vi "LoadDAQSettings.vi"(2 "error in":errorcluster, 4 "Current ExpState IN":T5={"error"={"status"=FALSE, "code"=0, "source"=""}, "Digitizer DAQmx Tasks"={"TaskArray"=[]}, "DAQ Settings"={"Channel Settings"=[], "Card Settings"=[]}, "Synchronization Settings"={"Synchronizer 0"="", "source terminal"="", "Synchronizer 1"="PXI1Slot2"}, "DAQ Data"=[], "Next Shot#"="", "System Message"="", "User Shot Notes"="", "Timing Settings"={"Timing Card Settings"=[], "Timing Channel Settings"=[]}, "Timing Tasks"={"TaskArray"=[]}, "Tree"="", "Time Card/Channels"=[2, 8], "DAQ Card/Channels"=[3, 8], "Program Version"="", "RIO Settings"={"Channel Settings"=[], "Card Settings"=[]}, "RIO References"={"Reference Array"=[]}, "RIO Data"={"RIO Deleaved Data"=[], "Raw Readout"=[]}, "RIO Card/Channels"=[3, 8], "DIO Channels"=0, "DIO Settings"={"DIO Channel Array"=[]}, "Tachometer Controls"={"Tach Calibration folder"=path "Z:/Data/Calibration/Tachometer", "PSU2 charging Voltage [kV]"=0.0, "PSU2 Counter"="", "PSU2 task"="PSU2", "PSU3 Counter"="", "PSU3 task"="", "PSU3 charging Voltage [kV]"=0.0}, "Global Settings"={"Initial Background Values"={"Reference Shot #"=0.0, "Background pressure [Torr]"=0.0, "Cryo temp [V]"=0.0, "Cryo temp [K]"=0.0, "Cryotemp Calibration File"=path ""}, "Gas Puffing"={"Gas A type"="N", "Gas B type"="N", "Gas C type"="N", "Gas A pressure [psi]"=0.0, "Gas B pressure [psi]"=0.0, "Gas C pressure [psi]"=0.0, "Innner Electrode"="", "Middle Electrode"="", "Outer Electrode"="", "Gas A bottle pressure [psi]"=0.0, "Gas B bottle pressure [psi]"=0.0, "Gas C bottle pressure [psi]"=0.0}, "PSU Voltages"={"Bias1 Voltage [V]"=0.0, "Bias2 Voltage [V]"=0.0, "PSU1 Voltage [V]"=0.0, "Puff-PSU1 CH1 Voltage [V]"=0.0, "Puff-PSU1 CH2 Voltage [V]"=0.0, "Puff-PSU1 CH3 Voltage [V]"=0.0}, "Scope Details"={"CH1"="", "CH2"="", "CH3"="", "CH4"="", "CH1 Ground State"="Grounded", "CH2 Ground State"="Grounded", "CH3 Ground State"="Grounded", "CH4 Ground State"="Grounded"}}, "Calibrations"={"CryoTemp"={"Comment"="", "X"=[], "Y"=[]}, "PSU2 Tach"={"Comment"="", "X"=[], "Y"=[]}, "PSU3 Tach"={"Comment"="", "X"=[], "Y"=[]}}} {"Global Settings"."Initial Background Values"."Cryo temp [K]" format="%#_4g"; "RIO Settings"."Card Settings"."Sample Rate" format="%#_3p"; "Timing Settings"."Timing Channel Settings"."FrontPanelTime" format="%.3p"; "Timing Settings"."Timing Channel Settings"."Pulse width (s)" format="%.3p"; "Timing Settings"."Timing Channel Settings"."Delay (s)" format="%.3p"; "DAQ Settings"."Card Settings"."Global Edge Type" items=["Rising"=10280, "Falling"=10171]; "DAQ Settings"."Card Settings"."Sample Rate" format="%#_3p"}, 5 "Tree DVR In":refnum<data-value>) -> (0 "error out":errorcluster, 1 "Digitizer Settings":T4 {"Card Settings"."Global Edge Type" items=["Rising"=10280, "Falling"=10171]; "Card Settings"."Sample Rate" format="%#_3p"})   [LabVIEW 2014]
uses:
  Controls/ExperimentStateCluster.ctl
  Controls/DigitizerSettingsChannelSettings.ctl
  Controls/DigitizerSettingsCardSettingsArray.ctl
  Controls/DigitizerSettingsCardSettings.ctl
  Controls/TimingSettings.ctl
  Controls/TimingCardSettings.ctl
  Controls/TimingChannelSettings.ctl
  Controls/RIOSettingsExperimentStateCluster.ctl
  Controls/RIOChannelSettingsArrayExperimentStateCluster.ctl
  Controls/RIOSettingsChannelSettings.ctl
  Controls/RIOSettingsCardSettingsArray.ctl
  Controls/RIOSettingsCardSettings.ctl
  <vilib>/userdefined/High Color/nirio_resource_hc.ctl
  Controls/RIOData.ctl
  Controls/DIOChannel.ctl
  Controls/TachometerControls.ctl
  Controls/Global Settings/GlobalSettings.ctl
  Controls/Global Settings/InitialBackgroundValues.ctl
  Controls/Global Settings/GasPuffing.ctl
  Controls/Global Settings/PSUVoltages.ctl
  Controls/Global Settings/ScopeDetails.ctl
  Controls/Calibrations/Calibrations.ctl
  Controls/Calibrations/CryoTemoCalibration.ctl
  Controls/Calibrations/PSU2TachCalibration.ctl
  Controls/Calibrations/PSU3TachCalibration.ctl
  <vilib>/MDSplus/Classes/Tree_Class/Tree.lvclass
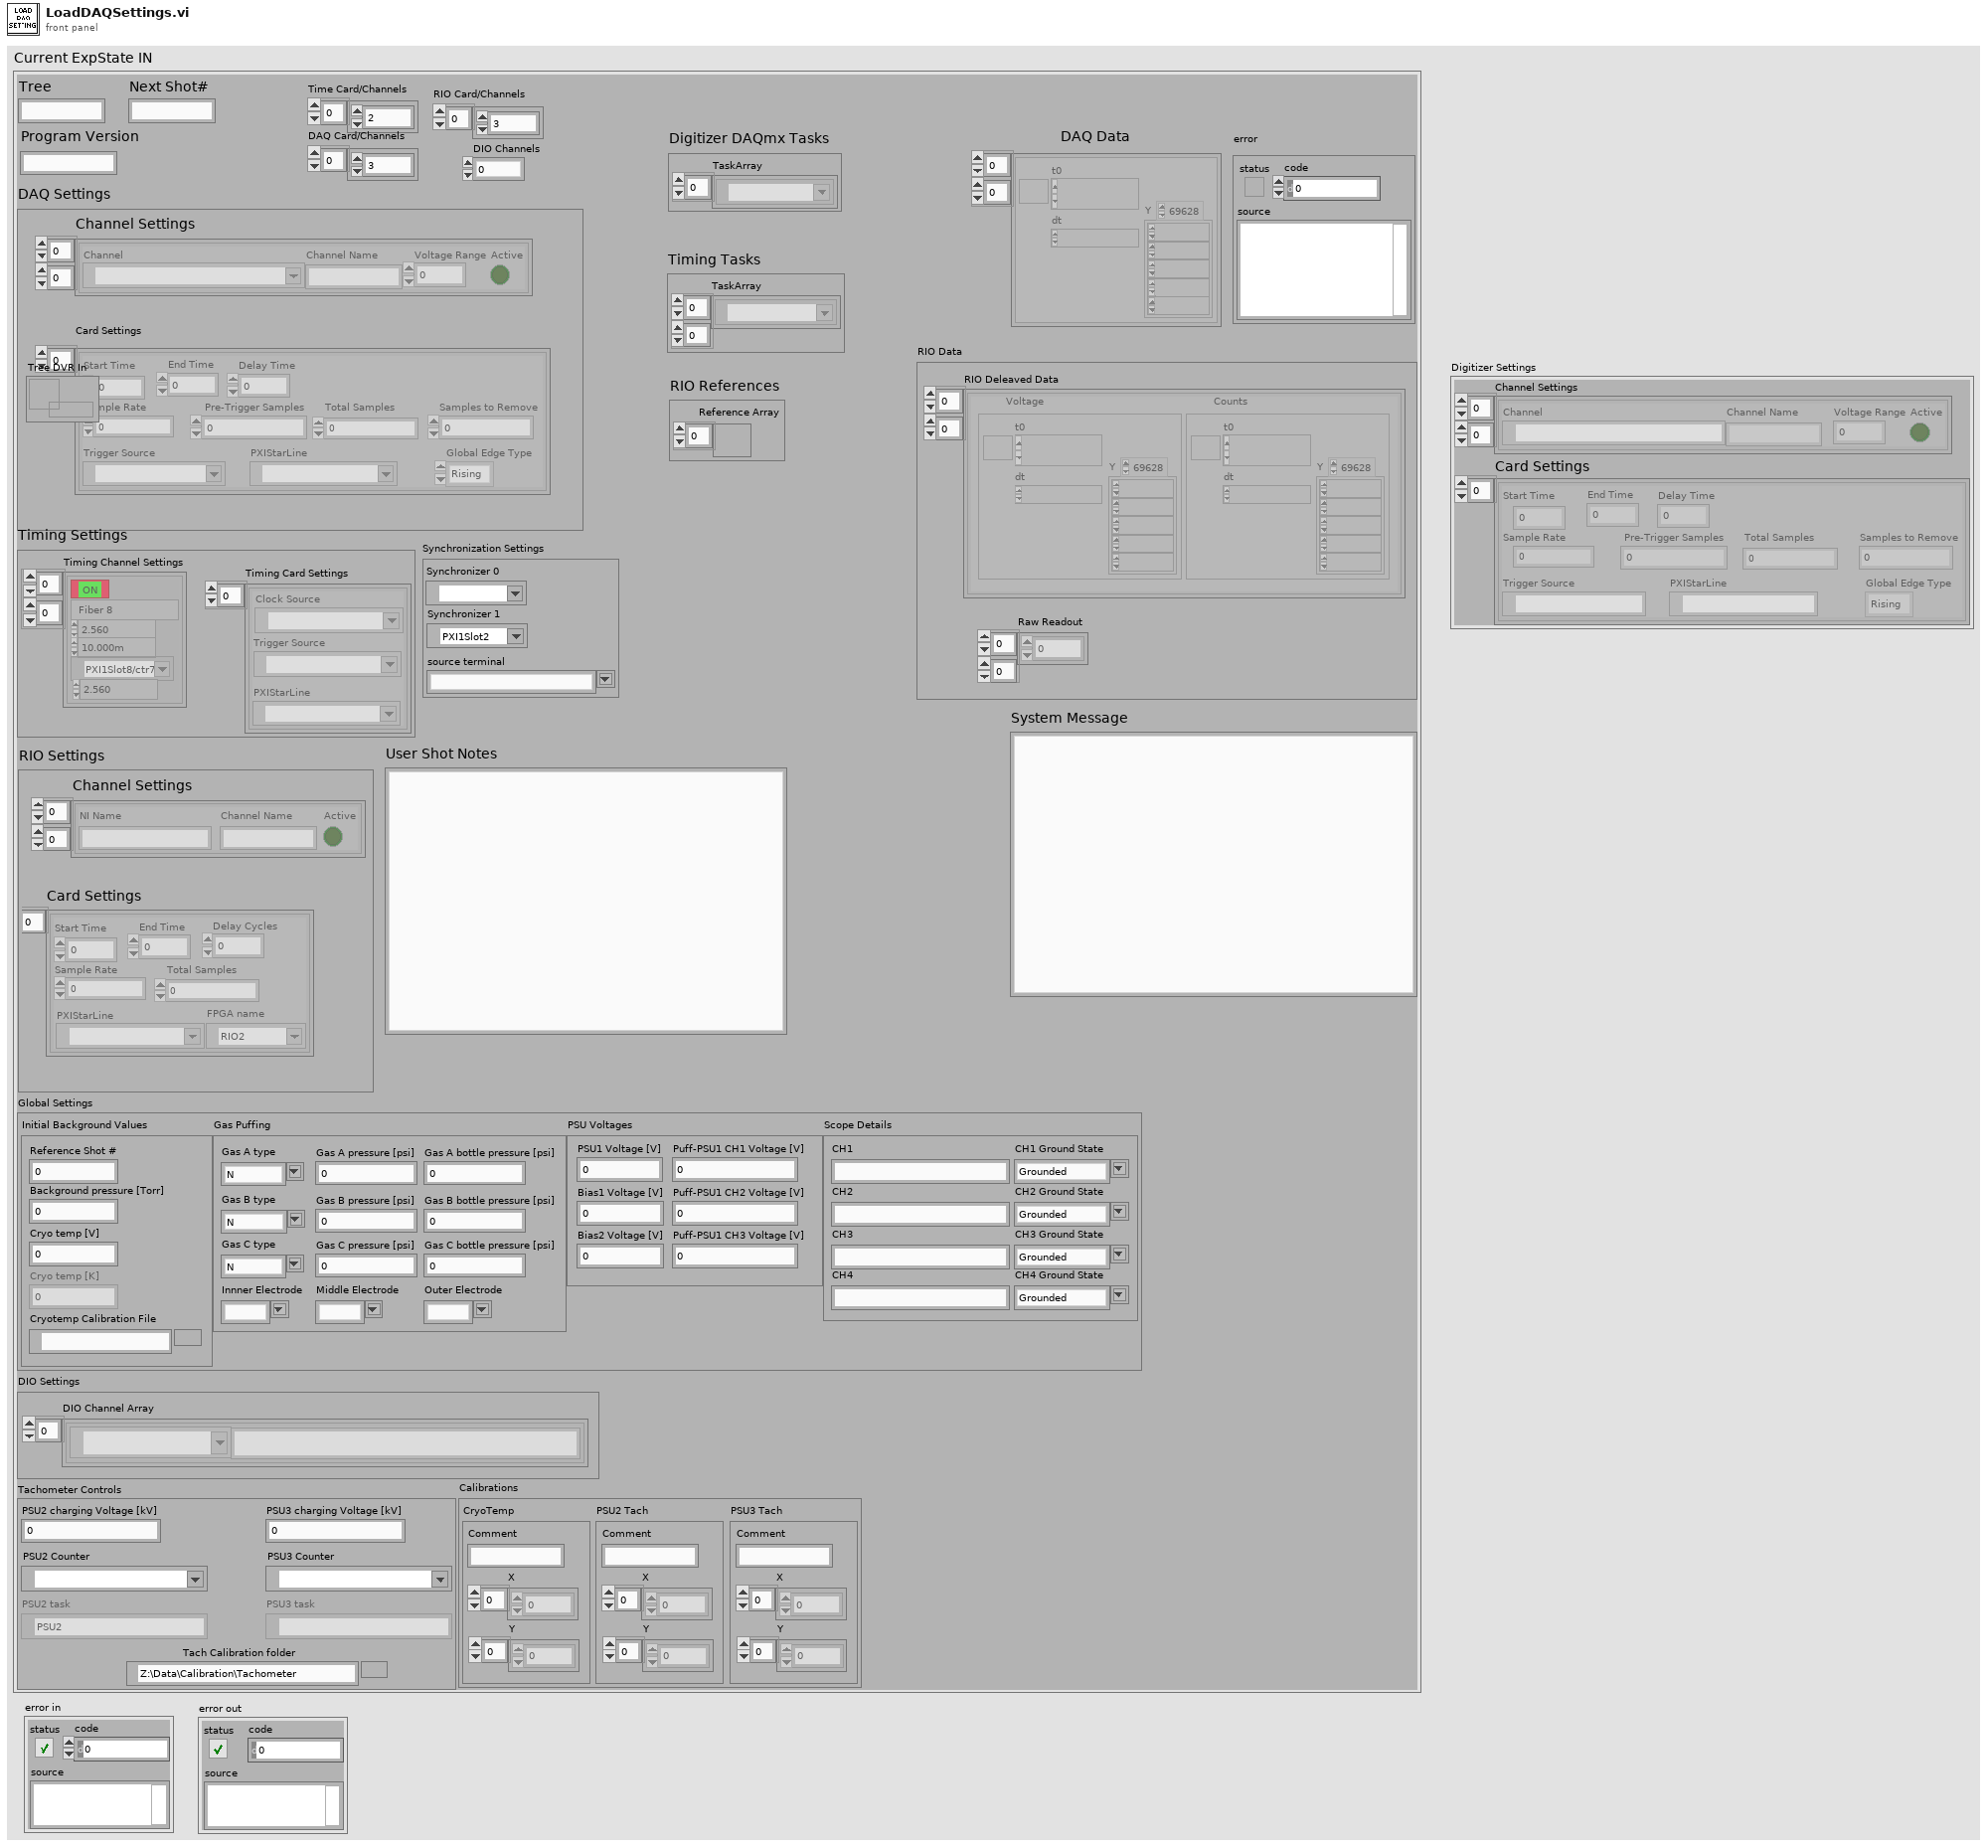
[diagram p1: front panel]
types:
  T1 = typedef "DigitizerSettingsChannelSettings.ctl" = cluster{"Channel":tag, "Channel Name":string, "Voltage Range":dbl, "Active":bool}
  T2 = typedef "DigitizerSettingsCardSettingsArray.ctl" = T3[]
  T3 = typedef "DigitizerSettingsCardSettings.ctl" = cluster{"Start Time":dbl, "End Time":dbl, "Sample Rate":dbl, " Pre-Trigger Samples":u32, "Total Samples":i32, "Samples to Remove":u32, "Trigger Source":tag, "Global Edge Type":i32, "PXIStarLine":tag, "Delay Time":dbl}
  T4 = cluster{"Channel Settings":T1[][], "Card Settings":T2}
  T5 = typedef "ExperimentStateCluster.ctl" = cluster{"error":errorcluster, "Digitizer DAQmx Tasks":cluster{"TaskArray":refnum<k21>[]}, "DAQ Settings":cluster{"Channel Settings":T1[][], "Card Settings":T2}, "Synchronization Settings":cluster{"Synchronizer 0":refnum<k15>, "source terminal":string, "Synchronizer 1":refnum<k15>}, "DAQ Data":waveform(dbl)[][], "Next Shot#":string, "System Message":string, "User Shot Notes":string, "Timing Settings":T6, "Timing Tasks":cluster{"TaskArray":refnum<k21>[][]}, "Tree":string, "Time Card/Channels":i32[], "DAQ Card/Channels":i32[], "Program Version":string, "RIO Settings":T9, "RIO References":cluster{"Reference Array":refnum<k20>[]}, "RIO Data":T15, "RIO Card/Channels":i32[], "DIO Channels":i32, "DIO Settings":cluster{"DIO Channel Array":T16[]}, "Tachometer Controls":T17, "Global Settings":T18, "Calibrations":T23}
  T6 = typedef "TimingSettings.ctl" = cluster{"Timing Card Settings":T7[], "Timing Channel Settings":T8[][]}
  T7 = typedef "TimingCardSettings.ctl" = cluster{"Trigger Source":tag, "Clock Source":tag, "PXIStarLine":tag}
  T8 = typedef "TimingChannelSettings.ctl" = cluster{"Delay (s)":dbl, "Pulse width (s)":dbl, "Active":bool, "Channel Name":string, "counter":tag, "FrontPanelTime":dbl}
  T9 = typedef "RIOSettingsExperimentStateCluster.ctl" = cluster{"Channel Settings":T10, "Card Settings":T12}
  T10 = typedef "RIOChannelSettingsArrayExperimentStateCluster.ctl" = T11[][]
  T11 = typedef "RIOSettingsChannelSettings.ctl" = cluster{"Channel Name":string, "Active":bool, "NI Name":string}
  T12 = typedef "RIOSettingsCardSettingsArray.ctl" = T13[]
  T13 = typedef "RIOSettingsCardSettings.ctl" = cluster{"Start Time":dbl, "End Time":dbl, "Sample Rate":dbl, "Total Samples":u64, "PXIStarLine":tag, "Delay Cycles":u64, "FPGA name":T14}
  T14 = typedef "nirio_resource_hc.ctl" = tag
  T15 = typedef "RIOData.ctl" = cluster{"RIO Deleaved Data":cluster{"Voltage":waveform(dbl), "Counts":waveform(i16)}[][], "Raw Readout":u64[][]}
  T16 = typedef "DIOChannel.ctl" = cluster{"Channel Name":string, "NI Name":tag}
  T17 = typedef "TachometerControls.ctl" = cluster{"Tach Calibration folder":path, "PSU2 charging Voltage [kV]":dbl, "PSU2 Counter":tag, "PSU2 task":refnum<k21>, "PSU3 Counter":tag, "PSU3 task":refnum<k21>, "PSU3 charging Voltage [kV]":dbl}
  T18 = typedef "GlobalSettings.ctl" = cluster{"Initial Background Values":T19, "Gas Puffing":T20, "PSU Voltages":T21, "Scope Details":T22}
  T19 = typedef "InitialBackgroundValues.ctl" = cluster{"Reference Shot #":dbl, "Background pressure [Torr]":dbl, "Cryo temp [V]":dbl, "Cryo temp [K]":dbl, "Cryotemp Calibration File":path}
  T20 = typedef "GasPuffing.ctl" = cluster{"Gas A type":string, "Gas B type":string, "Gas C type":string, "Gas A pressure [psi]":dbl, "Gas B pressure [psi]":dbl, "Gas C pressure [psi]":dbl, "Innner Electrode":string, "Middle Electrode":string, "Outer Electrode":string, "Gas A bottle pressure [psi]":dbl, "Gas B bottle pressure [psi]":dbl, "Gas C bottle pressure [psi]":dbl}
  T21 = typedef "PSUVoltages.ctl" = cluster{"Bias1 Voltage [V]":dbl, "Bias2 Voltage [V]":dbl, "PSU1 Voltage [V]":dbl, "Puff-PSU1 CH1 Voltage [V]":dbl, "Puff-PSU1 CH2 Voltage [V]":dbl, "Puff-PSU1 CH3 Voltage [V]":dbl}
  T22 = typedef "ScopeDetails.ctl" = cluster{"CH1":string, "CH2":string, "CH3":string, "CH4":string, "CH1 Ground State":string, "CH2 Ground State":string, "CH3 Ground State":string, "CH4 Ground State":string}
  T23 = typedef "Calibrations.ctl" = cluster{"CryoTemp":T24, "PSU2 Tach":T25, "PSU3 Tach":T26}
  T24 = typedef "CryoTemoCalibration.ctl" = cluster{"Comment":string, "X":dbl[], "Y":dbl[]}
  T25 = typedef "PSU2TachCalibration.ctl" = cluster{"Comment":string, "X":dbl[], "Y":dbl[]}
  T26 = typedef "PSU3TachCalibration.ctl" = cluster{"Comment":string, "X":dbl[], "Y":dbl[]}
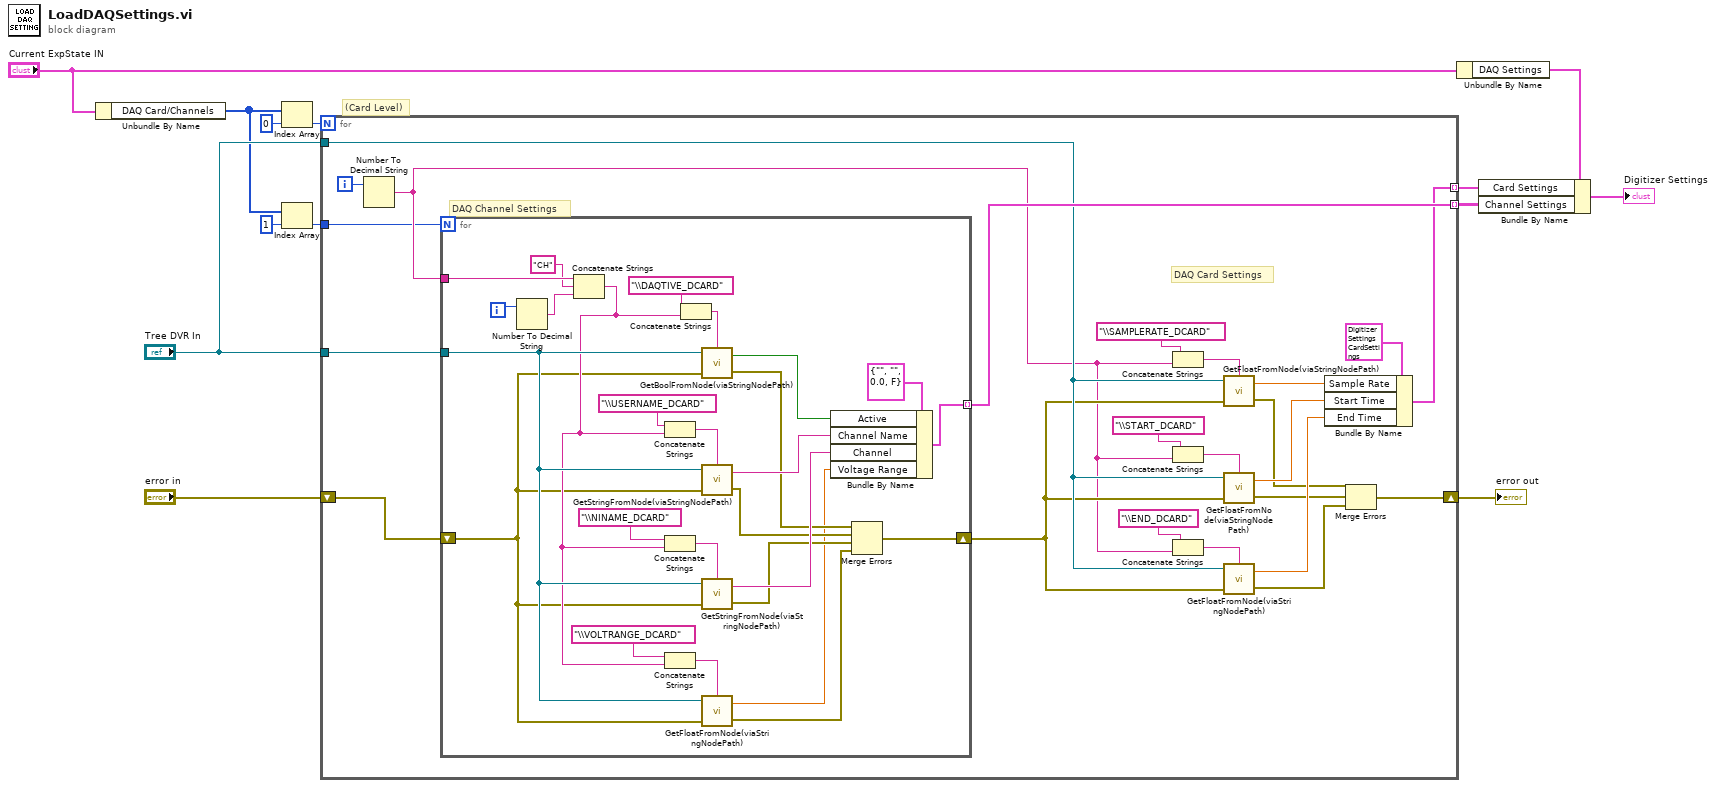
[diagram p0: block diagram]
diagram:
  # "(Card Level)"
  n1 = Unbundle By Name("Current ExpState IN") -> ("DAQ Card/Channels"=w1:i32[])
  n2 = Index Array(array=w1, index=0) -> (element=w12:i32)
  n3 = Index Array(array=w1, index=1) -> (element=w13:i32)
  n4 = for {
    N: w12 -> [_]
    tunnel: "Tree DVR In" -> [w35]
    shift-right: [w31] -> w5
    shift-left: "error in" -> [w27]
    tunnel: "Tree DVR In" -> [w33]
    tunnel: [w34] -> w3 mode=indexing
    tunnel: w13 -> [w28]
    tunnel: [w30] -> w4 mode=indexing
    i -> [w36]
    # "DAQ Card Settings"
    # "DAQ Channel Settings"
    n5 = Number To Decimal String(number=w36) -> (decimal integer string=w29:string)  [unwired: 1 in]
    n6 = for {
      N: w28 -> [_]
      tunnel: w35 -> [w59]
      tunnel: [w62] -> w34 mode=indexing
      tunnel: w29 -> [w60]
      shift-right: [w61] -> w32
      shift-left: w27 -> [w37]
      i -> [w58]
      n7 = Number To Decimal String(number=w58) -> (decimal integer string=w41:string)  [unwired: 1 in]
      n8 = Concatenate Strings(w60, "CH" ("string"), w41) -> (w39:string)
      n9 = Concatenate Strings("\\USERNAME_DCARD" ("string"), w39) -> (w53:string)
      n10 = Concatenate Strings("\\NINAME_DCARD" ("string"), w39) -> (w52:string)
      n11 = Concatenate Strings("\\VOLTRANGE_DCARD" ("string"), w39) -> (w51:string)
      n12 = Concatenate Strings("\\DAQTIVE_DCARD" ("string"), w39) -> (w54:string)
      n13 = call "GetBoolFromNode(viaStringNodePath).vi"("Path"=w54, "error in"=w37, "Tree DVR in"=w59) -> ("error out"=w47:errorcluster, "Bool Out"=w42:bool)  [unwired: 1 in]
      n14 = call "GetStringFromNode(viaStringNodePath).vi"("Path"=w53, "error in"=w37, "Tree DVR in"=w59) -> ("error out"=w46:errorcluster, "String out"=w49:string)  [unwired: 1 in]
      n15 = call "GetStringFromNode(viaStringNodePath).vi"("Path"=w52, "error in"=w37, "Tree DVR in"=w59) -> ("error out"=w45:errorcluster, "String out"=w48:string)  [unwired: 1 in]
      n16 = call "GetFloatFromNode(viaStringNodePath).vi"("Path"=w51, "error in"=w37, "Tree DVR in"=w59) -> ("error out"=w44:errorcluster, "Float64"=w43:dbl)  [unwired: 1 in]
      n17 = Bundle By Name(cluster=T1 {"Channel"="", "Channel Name"="", "Voltage Range"=0.0, "Active"=FALSE} ("Channel Setting"), "Active"=w42, "Channel Name"=w49, "Channel"=w48, "Voltage Range"=w43) -> (w62:T1)
      n18 = Merge Errors(w47, w46, w45, w44) -> (w61:errorcluster)
    }
    n19 = Concatenate Strings("\\SAMPLERATE_DCARD" ("string"), w29) -> (w25:string)
    n20 = Concatenate Strings("\\START_DCARD" ("string"), w29) -> (w21:string)
    n21 = Concatenate Strings("\\END_DCARD" ("string"), w29) -> (w24:string)
    n22 = call "GetFloatFromNode(viaStringNodePath).vi"("Path"=w25, "error in"=w32, "Tree DVR in"=w33) -> ("error out"=w17:errorcluster, "Float64"=w20:dbl)  [unwired: 1 in]
    n23 = call "GetFloatFromNode(viaStringNodePath).vi"("Path"=w21, "error in"=w32, "Tree DVR in"=w33) -> ("error out"=w16:errorcluster, "Float64"=w19:dbl)  [unwired: 1 in]
    n24 = call "GetFloatFromNode(viaStringNodePath).vi"("Path"=w24, "error in"=w32, "Tree DVR in"=w33) -> ("error out"=w15:errorcluster, "Float64"=w18:dbl)  [unwired: 1 in]
    n25 = Bundle By Name(cluster=T3 {"Start Time"=0.0, "End Time"=0.0, "Sample Rate"=0.0, " Pre-Trigger Samples"=0, "Total Samples"=0, "Samples to Remove"=0, "Trigger Source"="", "Global Edge Type"=10280, "PXIStarLine"="", "Delay Time"=0.0} ("Card Setting"), "Sample Rate"=w20, "Start Time"=w19, "End Time"=w18) -> (w30:T3)
    n26 = Merge Errors(w17, w16, w15) -> (w31:errorcluster)
  }
  "error out" <- w5
  n27 = Unbundle By Name("Current ExpState IN") -> ("DAQ Settings"=w9:T4)
  n28 = Bundle By Name(cluster=w9, "Card Settings"=w4, "Channel Settings"=w3) -> (→"Digitizer Settings":T4)
